vi "DriveReadEncoder.vi"(8 "error in":errorcluster, 11 "ModualNamePrefix":i32) -> (0 "error out":errorcluster, 2 "SWERVE_DRIVE_MODULE_POSITION":T1={"Distance"=0.0, "Angle"={"VALUE"=0.0, "COS"=1.0, "SIN"=0.0}, "P"=FALSE} {"Angle"."SIN" format="%13.4f"; "Angle"."COS" format="%13.4f"; "Angle"."VALUE" format="%13.4f"}, 3 "SWERVE_DRIVE_MODULE_STATE":T3={"Speed"=0.0, "Angle"={"VALUE"=0.0, "COS"=1.0, "SIN"=0.0}} {"Angle"."SIN" format="%13.4f"; "Angle"."COS" format="%13.4f"; "Angle"."VALUE" format="%13.4f"})   [LabVIEW 2023]
uses:
  <vilib>/Rock Robotics/Network Tables/NT Write Number.vi
  <vilib>/Rock Robotics/WPI/ThirdParty/JAS_Junk/TrajLib/Trajectory_Library.lvlib
  DriveGlobal.vi
  <vilib>/Rock Robotics/WPI/ThirdParty/Phoenix-LabVIEW/CANCoder/Get/CTRE_Phoenix_CANcoder_GetSensorData.vi
  <vilib>/Rock Robotics/WPI/ThirdParty/REV Robotics/REVLib/SubVI/Public/SPARK Get Encoder Status Position.vi
  <vilib>/Rock Robotics/WPI/ThirdParty/REV Robotics/REVLib/SubVI/Public/SPARK Get Encoder Status Velocity.vi
  <vilib>/Rock Robotics/WPI/ThirdParty/JAS_Junk/TrajLib/TypeDef/ROTATION2D.ctl
  <vilib>/Rock Robotics/WPI/ThirdParty/JAS_Junk/TrajLib/TypeDef/SWERVE_DRIVE_MODULE_STATE.ctl
  <vilib>/Rock Robotics/WPI/ThirdParty/JAS_Junk/TrajLib/TypeDef/SWERVE_DRIVE_MODULE_POSITION.ctl
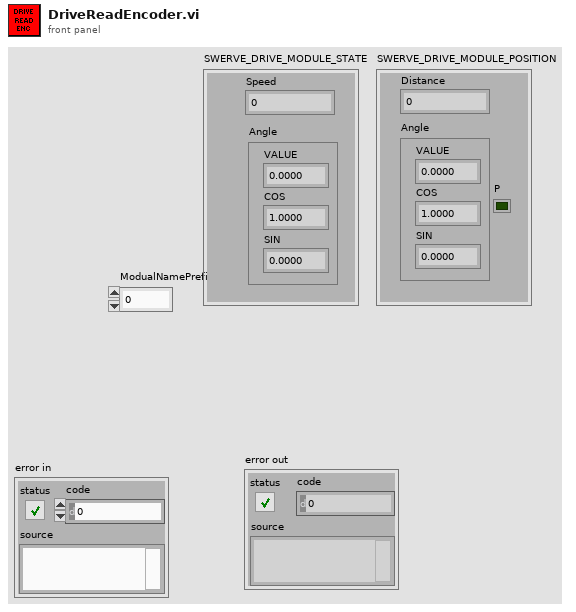
[diagram p1: front panel]
types:
  T1 = typedef "Trajectory_Library.lvlib/SWERVE_DRIVE_MODULE_POSITION.ctl" = cluster{"Distance":dbl, "Angle":T2, "P":bool}
  T2 = typedef "Trajectory_Library.lvlib/ROTATION2D.ctl" = cluster{"VALUE":dbl, "COS":dbl, "SIN":dbl}
  T3 = typedef "Trajectory_Library.lvlib/SWERVE_DRIVE_MODULE_STATE.ctl" = cluster{"Speed":dbl, "Angle":T2}
  T4 = typedef "WPI_MotorControlDeviceRef.ctl" = cluster{"DeviceStatus":errorcluster, "Type":T5, "PWM":cluster{"PWM Channel":T6, "DeadBand":T7}, "CAN":cluster{"Device Number":u8, "SetOutput VI Ref":variant, "GetOutput VI Ref":variant, "Enable VI Ref":variant, "Disable VI Ref":variant, "Data":variant}, "Invert":bool, "DIO PWM":cluster{"PWM \"Enable\" Channel":T6, "DIOChannel":T8, "PWM Rate":dbl}}
  T5 = typedef "WPI_MotorControlType.ctl" = enum16{"PWM", "CAN", "DIO PWM"}
  T6 = typedef "FPGA_DIOPWMChannel.ctl" = enum8{"PWM 0", "PWM 1", "PWM 2", "PWM 3", "PWM 4", "PWM 5", "PWM 6", "PWM 7", "PWM 8", "PWM 9", "PWM MXP 0", "PWM MXP 1", "PWM MXP 2", "PWM MXP 3", "PWM MXP 4", "PWM MXP 5", "PWM MXP 6", "PWM MXP 7", "PWM MXP 8", "PWM MXP 9", "Invalid"}
  T7 = typedef "WPI_PWMDeadband.ctl" = cluster{"Name":string, "maxPositivePwm":i32, "minPositivePwm":i32, "centerPwm":i32, "maxNegativePwm":i32, "minNegativePwm":i32, "angularRange":u16}
  T8 = typedef "FPGA_DIOChannel.ctl" = enum8{"DIO 0", "DIO 1", "DIO 2", "DIO 3", "DIO 4", "DIO 5", "DIO 6", "DIO 7", "DIO 8", "DIO 9", "DIO MXP 0", "DIO MXP 1", "DIO MXP 2", "DIO MXP 3", "DIO MXP 4", "DIO MXP 5", "DIO MXP 6", "DIO MXP 7", "DIO MXP 8", "DIO MXP 9", "DIO MXP 10", "DIO MXP 11", "DIO MXP 12", "DIO MXP 13", "DIO MXP 14", "DIO MXP 15", "SPI Port CS1", "SPI Port CS2", "SPI Port CS3", "SPI Port MISO", "SPI Port MOSI", "Invalid"}
  T9 = typedef "CTRE_Phoenix_CANcoder_DeviceRef.ctl" = cluster{"DeviceStatus":errorcluster, "Device Number":u8, "Handle":u64, "UsageFrame":u32, "Library Path":path}
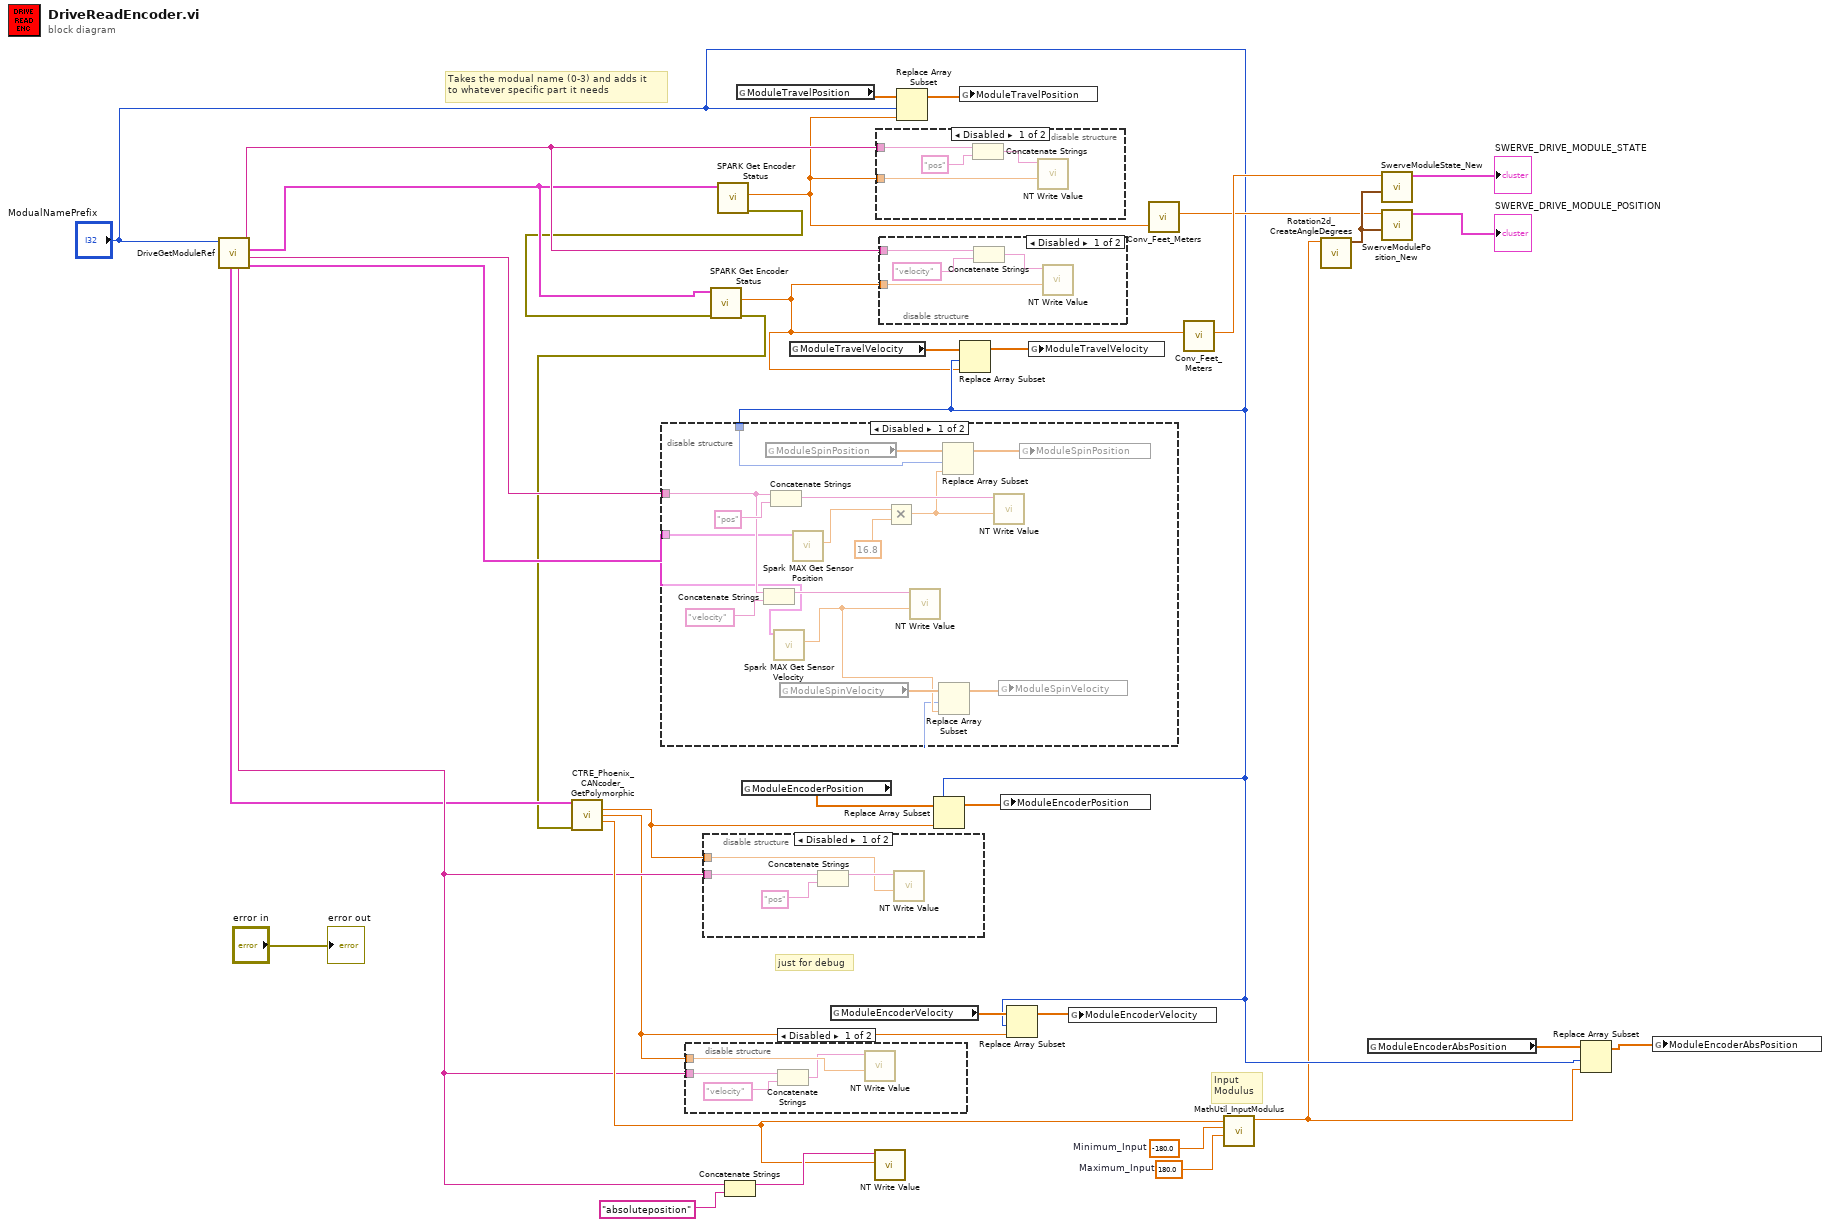
[diagram p0: block diagram]
diagram:
  w29 = -180.0  # Minimum_Input
  w28 = 180.0  # Maximum_Input
  # "Input\nModulus"
  # "just for debug"
  # "Takes the modual name (0-3) and adds it \nto whatever specific part it needs"
  n1 = call "DriveGetModuleRef.vi"("ModualNamePrefix"="ModualNamePrefix") -> ("SpinMot"=w20:T4, "SpinStr"=w22:string, "TravMot"=w4:T4, "TravStr"=w21:string, "EncStr"=w19:string, "EncDevice"=w18:T9)  [unwired: 5 in]
  n2 = disable-structure shown="Disabled" {
    disable-tunnel: w22 -> [w44 _]
    disable-tunnel: w20 -> [w43 _]
    disable-tunnel: "ModualNamePrefix" -> [w36 _]
    frame Disabled {
      n3 = Concatenate Strings(w44, "velocity" ("refnum name")) -> (w47:string)
      n4 = global read "DriveGlobal.vi" "ModuleSpinPosition"() -> (w42:dbl[])
      n5 = Concatenate Strings(w44, "pos" ("refnum name")) -> (w49:string)
      n6 = call <vilib>:"Spark MAX Get Sensor Velocity.vi"("MotorControlDevRef in"=w43) -> ("Sensor Velocity"=w37:dbl)  [unwired: 7 in, 3 out]
      n7 = global read "DriveGlobal.vi" "ModuleSpinVelocity"() -> (w39:dbl[])
      n8 = call <vilib>:"Spark MAX Get Sensor Position.vi"("MotorControlDevRef in"=w43) -> ("Sensor Position"=w46:dbl)  [unwired: 7 in, 3 out]
      n9 = Multiply(x=w46, y=16.8) -> (x*y=w40:dbl)
      n10 = call-poly <vilib>:"NT Write Value.vi"("value"=w37, "name"=w47) -> ()  [unwired: 9 in, 1 out]
      n11 = Replace Array Subset(array=w39, new element=w37, index=w36) -> (w38:dbl[])
      n12 = Replace Array Subset(array=w42, new element=w40, index=w36) -> (w41:dbl[])
      n13 = call-poly <vilib>:"NT Write Value.vi"("value"=w40, "name"=w49) -> ()  [unwired: 9 in, 1 out]
      n14 = global write "DriveGlobal.vi" "ModuleSpinVelocity"(w38) -> ()
      n15 = global write "DriveGlobal.vi" "ModuleSpinPosition"(w41) -> ()
    }
    frame Enabled {
    }
  }
  n16 = call-poly <vilib>:"SPARK Get Encoder Status.vi"("MotorControlDevRef in"=w4) -> ("error out"=w2:errorcluster, "Sensor Position"=w5:dbl)  [unwired: 7 in, 2 out]
  n17 = call-poly <vilib>:"SPARK Get Encoder Status.vi"("error in (no error)"=w2, "MotorControlDevRef in"=w4) -> ("error out"=w1:errorcluster, "Sensor Velocity"=w3:dbl)  [unwired: 6 in, 2 out]
  n18 = call-poly <vilib>:"CTRE_Phoenix_CANcoder_GetPolymorphic.vi"("CTRE_CANcoder_DeviceRef"=w18, "error in"=w1) -> ("Position"=w13:dbl, "Velocity"=w10:dbl, "Absolute Position"=w27:dbl)  [unwired: 9 in, 2 out]
  n19 = disable-structure shown="Disabled" {
    disable-tunnel: w19 -> [w54 _]
    disable-tunnel: w10 -> [w53 _]
    frame Disabled {
      n20 = Concatenate Strings(w54, "velocity" ("refnum name")) -> (w51:string)
      n21 = call-poly <vilib>:"NT Write Value.vi"("value"=w53, "name"=w51) -> ()  [unwired: 9 in, 1 out]
    }
    frame Enabled {
    }
  }
  n22 = disable-structure shown="Disabled" {
    disable-tunnel: w19 -> [w56 _]
    disable-tunnel: w13 -> [w55 _]
    frame Disabled {
      n23 = Concatenate Strings(w56, "pos" ("refnum name")) -> (w57:string)
      n24 = call-poly <vilib>:"NT Write Value.vi"("value"=w55, "name"=w57) -> ()  [unwired: 9 in, 1 out]
    }
    frame Enabled {
    }
  }
  n25 = Concatenate Strings(w19, "absoluteposition" ("refnum name")) -> (w33:string)
  n26 = global read "DriveGlobal.vi" "ModuleTravelPosition"() -> (w24:dbl[])
  n27 = global read "DriveGlobal.vi" "ModuleEncoderPosition"() -> (w15:dbl[])
  n28 = global read "DriveGlobal.vi" "ModuleTravelVelocity"() -> (w17:dbl[])
  n29 = global read "DriveGlobal.vi" "ModuleEncoderVelocity"() -> (w12:dbl[])
  n30 = call-poly <vilib>:"NT Write Value.vi"("value"=w27, "name"=w33) -> ()  [unwired: 9 in, 1 out]
  n31 = disable-structure shown="Disabled" {
    disable-tunnel: w21 -> [w60 _]
    disable-tunnel: w5 -> [w59 _]
    frame Disabled {
      n32 = Concatenate Strings(w60, "pos" ("refnum name")) -> (w61:string)
      n33 = call-poly <vilib>:"NT Write Value.vi"("value"=w59, "name"=w61) -> ()  [unwired: 9 in, 1 out]
    }
    frame Enabled {
    }
  }
  n34 = disable-structure shown="Disabled" {
    disable-tunnel: w21 -> [w64 _]
    disable-tunnel: w3 -> [w63 _]
    frame Disabled {
      n35 = Concatenate Strings(w64, "velocity" ("refnum name")) -> (w65:string)
      n36 = call-poly <vilib>:"NT Write Value.vi"("value"=w63, "name"=w65) -> ()  [unwired: 9 in, 1 out]
    }
    frame Enabled {
    }
  }
  n37 = Replace Array Subset(array=w24, new element=w5, index="ModualNamePrefix") -> (w23:dbl[])
  n38 = Replace Array Subset(array=w15, new element=w13, index="ModualNamePrefix") -> (w14:dbl[])
  n39 = global write "DriveGlobal.vi" "ModuleTravelPosition"(w23) -> ()
  n40 = Replace Array Subset(array=w17, new element=w3, index="ModualNamePrefix") -> (w16:dbl[])
  n41 = global write "DriveGlobal.vi" "ModuleEncoderPosition"(w14) -> ()
  n42 = Replace Array Subset(array=w12, new element=w10, index="ModualNamePrefix") -> (w11:dbl[])
  n43 = global write "DriveGlobal.vi" "ModuleTravelVelocity"(w16) -> ()
  n44 = global write "DriveGlobal.vi" "ModuleEncoderVelocity"(w11) -> ()
  n45 = call <vilib>:"Conv_Feet_Meters.vi"("Feet"=w5) -> ("Meters"=w25:dbl)  [unwired: 10 in]
  n46 = call <vilib>:"Conv_Feet_Meters.vi"("Feet"=w3) -> ("Meters"=w26:dbl)  [unwired: 10 in]
  n47 = call <vilib>:"MathUtil_InputModulus.vi"("Maximum_Input"=w28, "Minimum_Input"=w29, "Input"=w27) -> ("modulus"=w6:dbl)  [unwired: 8 in]
  n48 = call <vilib>:"Rotation2d_CreateAngleDegrees.vi"("Angle_Degrees"=w6) -> ("ROTATION"=w32:T2)  [unwired: 10 in]
  n49 = global read "DriveGlobal.vi" "ModuleEncoderAbsPosition"() -> (w9:dbl[])
  n50 = call <vilib>:"SwerveModuleState_New.vi"("ROTATION"=w32, "Speed"=w26) -> ("SWERVE_DRIVE_MODULE_STATE"=→"SWERVE_DRIVE_MODULE_STATE":T3)  [unwired: 9 in]
  n51 = call <vilib>:"SwerveModulePosition_New.vi"("ROTATION"=w32, "Distance"=w25) -> ("SWERVE_DRIVE_MODULE_POSITION"=→"SWERVE_DRIVE_MODULE_POSITION":T1)  [unwired: 9 in]
  n52 = Replace Array Subset(array=w9, new element=w6, index="ModualNamePrefix") -> (w8:dbl[])
  n53 = global write "DriveGlobal.vi" "ModuleEncoderAbsPosition"(w8) -> ()
  "error out" <- "error in"
